vi "Add FIU Card.vi"(8 "error in (no error)":errorcluster, 11 "Node Ptr":u64 format="%.0x") -> (0 "error out":errorcluster)   [LabVIEW 2014, in "SLSC configuration System Explorer.lvlib"]
uses:
  SLSC configuration System Explorer.lvlib
  Shared/Constants.vi
  Shared/SLSC configuration Shared.lvlib
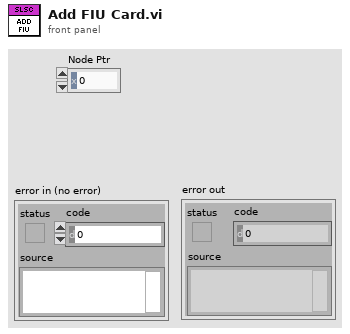
[diagram p1: front panel]
types:
  T1 = typedef "SLSC configuration Shared.lvlib/Card Position.ctl" = cluster{"Rack #":u8, "Slot #":T2}
  T2 = typedef "SLSC configuration Shared.lvlib/Slot #.ctl" = u8
  T3 = typedef "Custom Device API.lvlib/Custom Device Item Ref.ctl" = u64
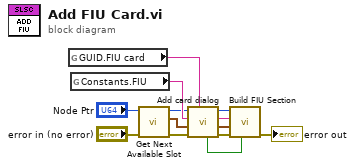
[diagram p0: block diagram]
diagram:
  n1 = global read "Constants.vi" "GUID.FIU card"() -> (w1:string)
  n2 = global read "Constants.vi" "Constants.FIU"() -> (w9:string)
  n3 = call "Get Next Available Slot.vi"("error in (no error)"="error in (no error)", "Device Ref in"="Node Ptr") -> ("error out"=w5:errorcluster, "Next Open Slot"=w4:T1, "Device Ref out"=w2:T3)  [unwired: 7 in]
  n4 = call "Add card dialog.vi"("Card GUID"=w1, "error in (no error)"=w5, "Card Position"=w4, "Card Type in"=w9, "Node Ptr"=w2) -> ("error out"=w11:errorcluster, "Card Position out"=w10:T1, "Name out"=w12:string, "Node Ptr out"=w13:u64, "Cancelled?"=w7:bool)  [unwired: 2 in]
  n5 = call "Build FIU Section.vi"("Cancelled?"=w7, "error in (no error)"=w11, "Card Position in"=w10, "Name in"=w12, "Node Ptr in"=w13) -> ("error out"=→"error out":errorcluster)  [unwired: 6 in]
